vi "Solution part 2.vi"() -> ()   [LabVIEW 2020]
uses:
  <vilib>/Utility/file.llb/Read Delimited Spreadsheet (I64).vi
panel:
  out "all geq0?":bool
  out "result":i64
  in  "data?":bool
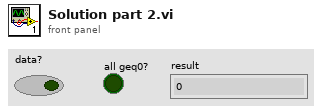
[diagram p1: front panel]
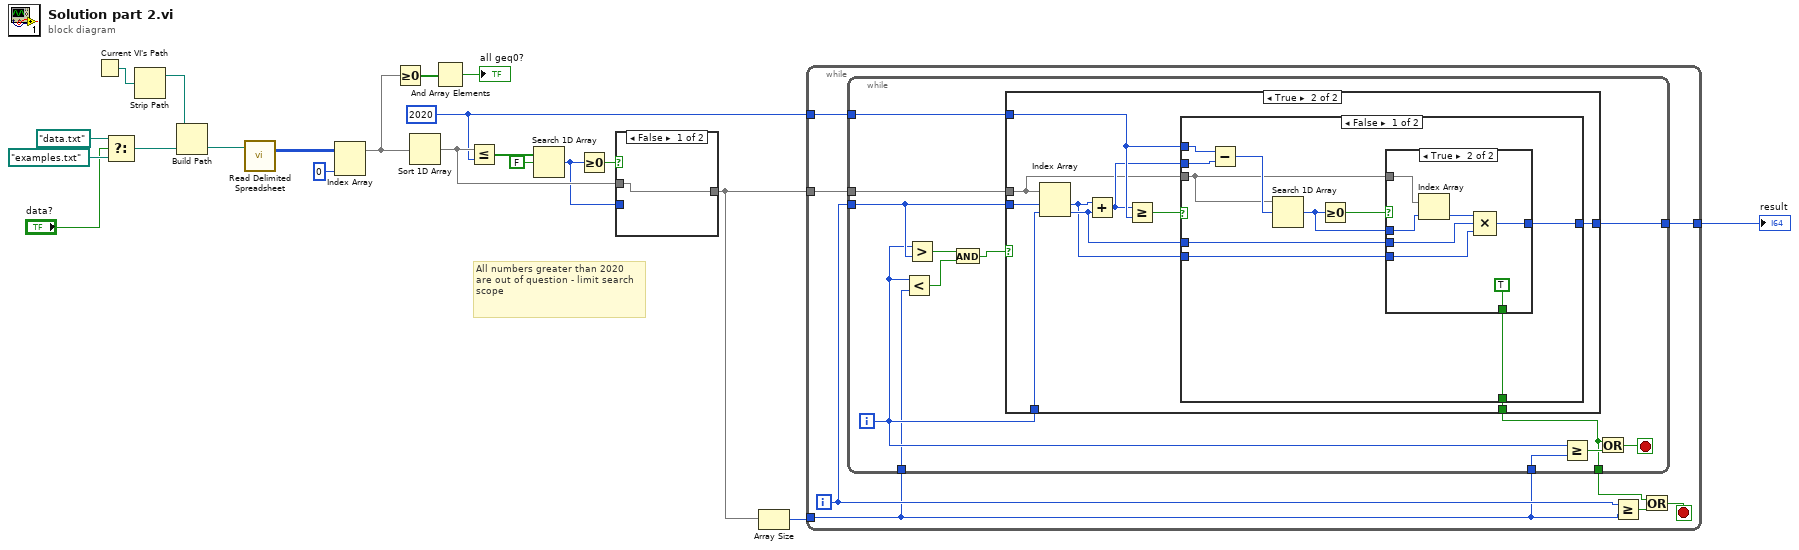
[diagram p0: block diagram]
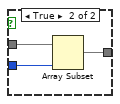
[diagram p2: hidden frame]
diagram:
  w6 = i64 2020 ("disabled index (col)")
  # "All numbers greater than 2020\nare out of question - limit search scope"
  n1 = Current VI's Path() -> (path=w17:path)
  n2 = Select(t=path "data.txt", s="data?", f=path "examples.txt") -> (s? t:f=w18:path)
  n3 = Strip Path(path=w17) -> (stripped path=w16:path)  [unwired: 1 out]
  n4 = Build Path(base path=w16, name or relative path=w18) -> (appended path=w15:path)
  n5 = call-poly <vilib>:"Read Delimited Spreadsheet.vi"("file path (dialog if empty)"=w15) -> ("all rows"=w14:i64[][])  [unwired: 9 in, 5 out]
  n6 = Index Array(array=w14, index (col)=0 ("disabled index (col)")) -> (element=w9:i64[])  [unwired: 1 in]
  n7 = Greater Or Equal To 0?(x=w9) -> (x >= 0?=w8:bool[])
  n8 = Sort 1D Array(array=w9) -> (sorted array=w10:i64[])
  n9 = And Array Elements(Boolean array=w8) -> (logical AND=→"all geq0?":bool)
  n10 = Less Or Equal?(x=w10, y=w6) -> (x <= y?=w12:bool[])
  n11 = Search 1D Array(1D array=w12, element=FALSE) -> (index of element=w2:i32)  [unwired: 1 in]
  n12 = Greater Or Equal To 0?(x=w2) -> (x >= 0?=w3:bool)
  n13 = case shown="False" w3 {
    tunnel: w10 -> [w22 w25]
    tunnel: [w22 w24] -> w1
    tunnel: w2 -> [_ w23]
    frame False {
    }
    frame True {
      n14 = Array Subset(array=w25, length=w23) -> (w24:i64[])  [unwired: 1 in]
    }
  }
  n15 = Array Size(array=w1) -> (size(s)=w4:i32)
  n16 = while {
    tunnel: w1 -> [w33]
    tunnel: w6 -> [w32]
    tunnel: [w31] -> w5
    tunnel: w4 -> [w26]
    i -> [w28]
    stop <- w29 stop-if-true
    n17 = while {
      tunnel: w33 -> [w46]
      tunnel: w28 -> [w43]
      tunnel: w32 -> [w45]
      tunnel: [w42] -> w31
      tunnel: w26 -> [w39]
      tunnel: [w38] -> w27
      tunnel: w26 -> [w36]
      i -> [w37]
      stop <- w40 stop-if-true
      n18 = Less?(x=w37, y=w36) -> (x < y?=w34:bool)
      n19 = Greater?(x=w37, y=w43) -> (0:w44:bool)
      n20 = And(x=w44, y=w34) -> (x .and. y?=w35:bool)
      n21 = case shown="True" w35 {
        tunnel: w46 -> [_ w51]
        tunnel: w43 -> [_ w56]
        tunnel: w37 -> [_ w55]
        tunnel: w45 -> [_ w53]
        tunnel: [_ w48] -> w42
        tunnel: [_ w47] -> w38
        frame False {
        }
        frame True {
          n22 = Index Array(array=w51, index #1=w56, index #2=w55) -> (element #1=w49:i64, element #2=w50:i64)
          n23 = Add(x=w49, y=w50) -> (x+y=w52:i64)
          n24 = Greater Or Equal?(x=w52, y=w53) -> (x >= y?=w54:bool)
          n25 = case shown="False" w54 {
            tunnel: w53 -> [w66 _]
            tunnel: w52 -> [w65 _]
            tunnel: w51 -> [w61 _]
            tunnel: w50 -> [w60 _]
            tunnel: w49 -> [w59 _]
            tunnel: [w58 _] -> w48
            tunnel: [w57 _] -> w47
            frame False {
              n26 = Subtract(x=w66, y=w65) -> (x-y=w64:i64)
              n27 = Search 1D Array(1D array=w61, element=w64) -> (index of element=w62:i32)  [unwired: 1 in]
              n28 = Greater Or Equal To 0?(x=w62) -> (x >= 0?=w63:bool)
              n29 = case shown="True" w63 {
                tunnel: w62 -> [w67 w74]
                tunnel: w61 -> [_ w73]
                tunnel: w60 -> [_ w71]
                tunnel: w59 -> [_ w70]
                tunnel: [w67 w69] -> w58
                tunnel: [_ TRUE] -> w57
                frame False {
                }
                frame True {
                  n30 = Index Array(array=w73, index=w74) -> (element=w72:i64)
                  n31 = Compound Arithmetic op=MULTIPLY(w72, w71, w70) -> (w69:i64)
                }
              }
            }
            frame True {
            }
          }
        }
      }
      n32 = Greater Or Equal?(x=w37, y=w39) -> (x >= y?=w41:bool)
      n33 = Or(x=w38, y=w41) -> (x .or. y?=w40:bool)
    }
    n34 = Greater Or Equal?(x=w28, y=w26) -> (x >= y?=w30:bool)
    n35 = Or(x=w27, y=w30) -> (x .or. y?=w29:bool)
  }
  "result" <- w5
